vi "Coloured_Dot_Plotting.vi"(1 "JobVectorDirectory":path, 2 "Data":string[][](array[string]), 3 "Template Filename":path, 4 "Channel Names":string[](array[string])) -> ()   [LabVIEW 2015]
uses:
  Controls/Group_Binning.ctl
  Data_File_Type.ctl
panel:
  in  "Moving Z":u16(ring) items=["FF (C) X Position X (mm)", "FF (C) Y Position Y (mm)", "FF (C) Z Position Z (mm)", "FF (C) Mean C", "FF (C) Variance c^2", "EnFlo_Tunnel Source_Pos X", "EnFlo_Tunnel Source_Pos Y", "EnFlo_Tunnel Source_Pos Z", "EnFlo_Tunnel Reference Velocity", "GMU Trace Meas Q", "Multi Run Start Time", "Delta_x", "Delta_y", "Delta_z", "R", "User Comments", "EnFlo_Tunnel Source_Pos X_Model", "EnFlo_Tunnel Source_Pos Y_Model"]
  in  "Moving Y":u16(ring) items=["FF (C) X Position X (mm)", "FF (C) Y Position Y (mm)", "FF (C) Z Position Z (mm)", "FF (C) Mean C", "FF (C) Variance c^2", "EnFlo_Tunnel Source_Pos X", "EnFlo_Tunnel Source_Pos Y", "EnFlo_Tunnel Source_Pos Z", "EnFlo_Tunnel Reference Velocity", "GMU Trace Meas Q", "Multi Run Start Time", "Delta_x", "Delta_y", "Delta_z", "R", "User Comments", "EnFlo_Tunnel Source_Pos X_Model", "EnFlo_Tunnel Source_Pos Y_Model"]
  in  "Moving X":u16(ring) items=["FF (C) X Position X (mm)", "FF (C) Y Position Y (mm)", "FF (C) Z Position Z (mm)", "FF (C) Mean C", "FF (C) Variance c^2", "EnFlo_Tunnel Source_Pos X", "EnFlo_Tunnel Source_Pos Y", "EnFlo_Tunnel Source_Pos Z", "EnFlo_Tunnel Reference Velocity", "GMU Trace Meas Q", "Multi Run Start Time", "Delta_x", "Delta_y", "Delta_z", "R", "User Comments", "EnFlo_Tunnel Source_Pos X_Model", "EnFlo_Tunnel Source_Pos Y_Model"]
  in  "Scalar":u16(ring) items=["FF (C) X Position X (mm)", "FF (C) Y Position Y (mm)", "FF (C) Z Position Z (mm)", "FF (C) Mean C", "FF (C) Variance c^2", "EnFlo_Tunnel Source_Pos X", "EnFlo_Tunnel Source_Pos Y", "EnFlo_Tunnel Source_Pos Z", "EnFlo_Tunnel Reference Velocity", "GMU Trace Meas Q", "Multi Run Start Time", "Delta_x", "Delta_y", "Delta_z", "R", "User Comments", "EnFlo_Tunnel Source_Pos X_Model", "EnFlo_Tunnel Source_Pos Y_Model"]
  in  "Fixed Z":u16(ring) items=["FF (C) X Position X (mm)", "FF (C) Y Position Y (mm)", "FF (C) Z Position Z (mm)", "FF (C) Mean C", "FF (C) Variance c^2", "EnFlo_Tunnel Source_Pos X", "EnFlo_Tunnel Source_Pos Y", "EnFlo_Tunnel Source_Pos Z", "EnFlo_Tunnel Reference Velocity", "GMU Trace Meas Q", "Multi Run Start Time", "Delta_x", "Delta_y", "Delta_z", "R", "User Comments", "EnFlo_Tunnel Source_Pos X_Model", "EnFlo_Tunnel Source_Pos Y_Model"]
  in  "Fixed Y":u16(ring) items=["FF (C) X Position X (mm)", "FF (C) Y Position Y (mm)", "FF (C) Z Position Z (mm)", "FF (C) Mean C", "FF (C) Variance c^2", "EnFlo_Tunnel Source_Pos X", "EnFlo_Tunnel Source_Pos Y", "EnFlo_Tunnel Source_Pos Z", "EnFlo_Tunnel Reference Velocity", "GMU Trace Meas Q", "Multi Run Start Time", "Delta_x", "Delta_y", "Delta_z", "R", "User Comments", "EnFlo_Tunnel Source_Pos X_Model", "EnFlo_Tunnel Source_Pos Y_Model"]
  in  "Fixed X":u16(ring) items=["FF (C) X Position X (mm)", "FF (C) Y Position Y (mm)", "FF (C) Z Position Z (mm)", "FF (C) Mean C", "FF (C) Variance c^2", "EnFlo_Tunnel Source_Pos X", "EnFlo_Tunnel Source_Pos Y", "EnFlo_Tunnel Source_Pos Z", "EnFlo_Tunnel Reference Velocity", "GMU Trace Meas Q", "Multi Run Start Time", "Delta_x", "Delta_y", "Delta_z", "R", "User Comments", "EnFlo_Tunnel Source_Pos X_Model", "EnFlo_Tunnel Source_Pos Y_Model"]
  in  "OK Button":bool
  in  "Row Selector":i32(listbox)=1
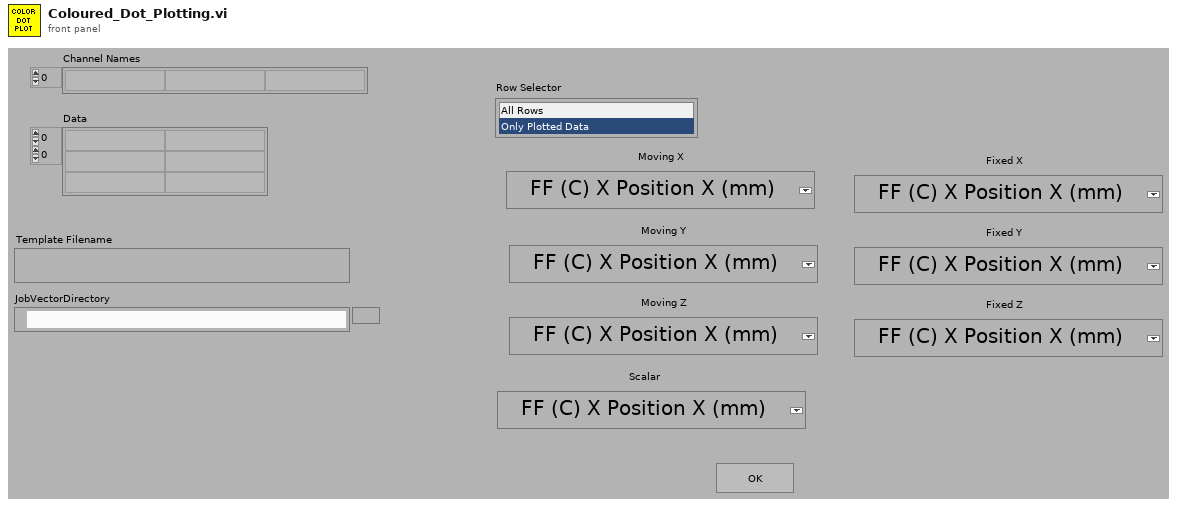
[diagram p1: front panel]
types:
  T1 = typedef "Data_File_Type.ctl" = enum16{"Read All File Types", "Results Files Only", "Raw Data Files Only", "Calibration Files Only", "Gas Desk Files Only", "Old Results Files Only", "Tabulated Data Files Only"}
  T2 = enum16{"Show only data summary", "Show data summary", "No data summary"}
  T3 = typedef "Group_Binning.ctl" = cluster{"Index":i32, "Tolerance":dbl, "Precision":string}
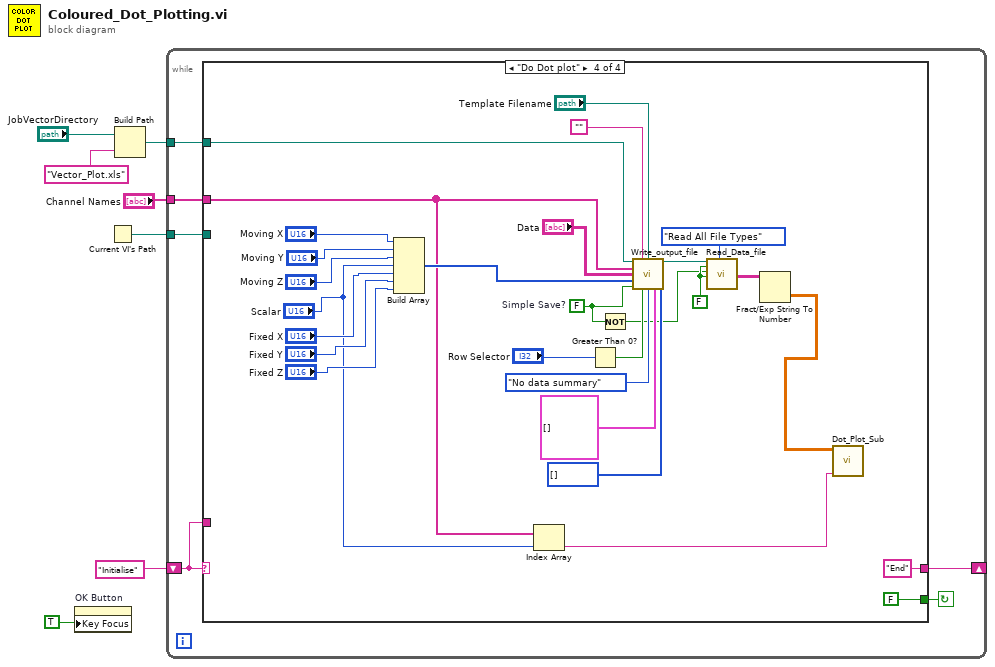
[diagram p0: block diagram]
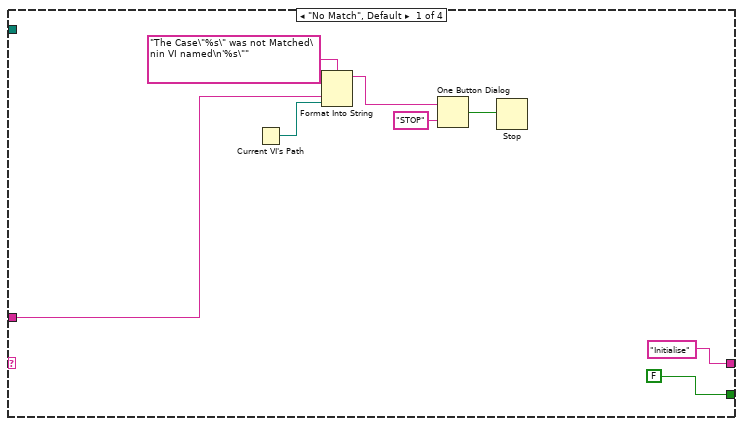
[diagram p2: hidden frame]
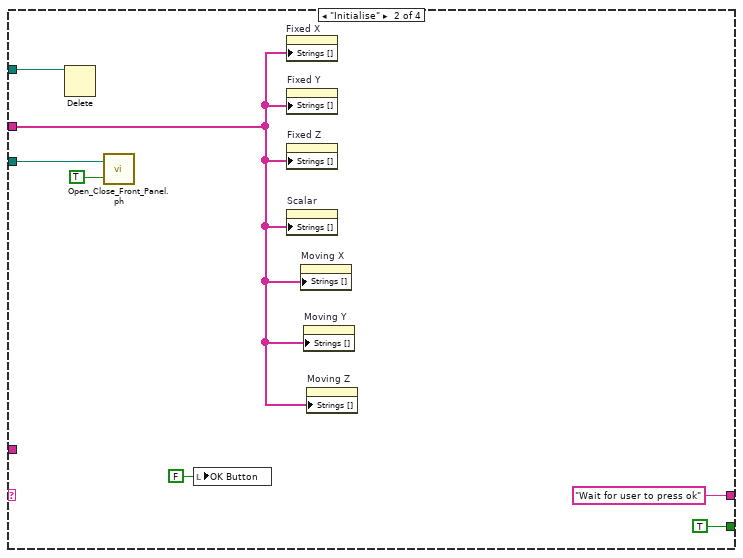
[diagram p3: hidden frame]
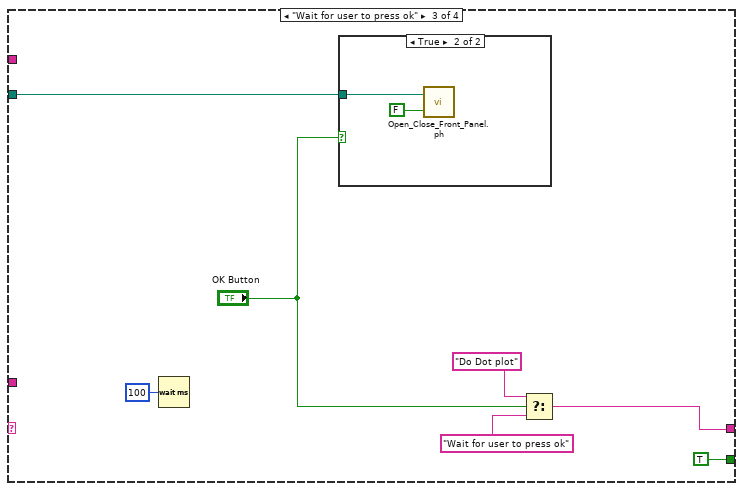
[diagram p4: hidden frame]
diagram:
  n1 = property on="OK Button" class="Bool (strict)"("Key Focus"=TRUE) -> ()  [unwired: 2 in, 2 out]
  n2 = Current VI's Path() -> (path=w6:path)
  n3 = Build Path(base path="JobVectorDirectory", name or relative path="Vector_Plot.xls") -> (appended path=w1:path)
  n4 = while {
    shift-left: "Initialise" -> [w11]
    shift-right: [w12] -> _
    tunnel: w6 -> [w10]
    tunnel: "Channel Names" -> [w9]
    tunnel: w1 -> [w8]
    stop <- w13 continue-if-true
    n5 = case shown="\"Do Dot plot\"" w11 {
      tunnel: [FALSE TRUE TRUE FALSE] -> w13
      tunnel: ["Initialise" "Wait for user to press ok" w34 "End" ("t")] -> w12
      tunnel: w11 -> [w16 _ _ _]
      tunnel: w10 -> [_ w26 w29 _]
      tunnel: w9 -> [_ w22 _ w43]
      tunnel: w8 -> [_ w23 _ w53]
      frame "No Match", Default {
        n6 = Current VI's Path() -> (path=w15:path)
        n7 = Format Into String(format string="The Case\"%s\" was not Matched\nin VI named\n'%s\"" ("Format String"), w16, w15) -> (resulting string=w19:string)  [unwired: 2 in, 1 out]
        n8 = One Button Dialog(message=w19, button name ("OK")="STOP") -> (true=w17:bool)
        n9 = Stop(stop? (T)=w17) -> ()
      }
      frame "Initialise" {
        n10 = Delete(path (use dialog)=w23) -> ()  [unwired: 1 in, 6 out]
        n11 = call "Open_Close_Front_Panel.ph.vi"("Front Panel Window:Open"=TRUE, "VI path"=w26) -> ()  [unwired: 2 out]
        n12 = local write "OK Button"(FALSE ("OK Button")) -> ()
        n13 = property on="Fixed X" class="Ring (strict)"("Strings []"=w22) -> ()  [unwired: 2 in, 2 out]
        n14 = property on="Fixed Y" class="Ring (strict)"("Strings []"=w22) -> ()  [unwired: 2 in, 2 out]
        n15 = property on="Fixed Z" class="Ring (strict)"("Strings []"=w22) -> ()  [unwired: 2 in, 2 out]
        n16 = property on="Scalar" class="Ring (strict)"("Strings []"=w22) -> ()  [unwired: 2 in, 2 out]
        n17 = property on="Moving X" class="Ring (strict)"("Strings []"=w22) -> ()  [unwired: 2 in, 2 out]
        n18 = property on="Moving Y" class="Ring (strict)"("Strings []"=w22) -> ()  [unwired: 2 in, 2 out]
        n19 = property on="Moving Z" class="Ring (strict)"("Strings []"=w22) -> ()  [unwired: 2 in, 2 out]
      }
      frame "Wait for user to press ok" {
        n20 = Wait (ms)(milliseconds to wait=u32 100) -> ()  [unwired: 1 out]
        n21 = case shown="True" "OK Button" {
          tunnel: w29 -> [_ w36]
          frame False {
          }
          frame True {
            n22 = call "Open_Close_Front_Panel.ph.vi"("Front Panel Window:Open"=FALSE, "VI path"=w36) -> ()  [unwired: 2 out]
          }
        }
        n23 = Select(t="Do Dot plot", s="OK Button", f="Wait for user to press ok") -> (s? t:f=w34:string)
      }
      frame "Do Dot plot" {
        w56 = FALSE ("Read Channel Names only")
        w40 = FALSE  # Simple Save?
        n24 = Build Array("Moving X", "Moving Y", "Moving Z", "Scalar", "Fixed X", "Fixed Y", "Fixed Z") -> (w44:u16[])
        n25 = Index Array(array=w43, index="Scalar") -> (element=w41:string)
        n26 = Greater Than 0?(x="Row Selector") -> (x > 0?=w59:bool)
        n27 = Not(x=w40) -> (.not. x?=w39:bool)
        n28 = call "Write_output_file.vi"("Output filename"=w53, "Header"="", "Template Filename"="Template Filename", "Channel Names"=w43, "Data"="Data", "Desired Columns"=w44, "Simple Save?"=w40, "Save Plotted rows only?"=w59, "Summarise mode"=T2."No data summary", "Grouping info"=T3[] [], "Channels to Tabulate in header"=i32[] []) -> ("Output filename Out"=w51:path)  [unwired: 1 in, 3 out]
        n29 = call "Read_Data_file.vi"("Results file"=w51, "Read Channel Names only"=w56, "Delete First Rows?"=w39, "Add Extra Channels?"=w56, "Desired File Types"=Data_File_Type."Read All File Types") -> ("Channel Values Out"=w54:string[][])  [unwired: 1 in, 13 out]
        n30 = Fract/Exp String To Number(string=w54) -> (number=w38:dbl[][])  [unwired: 4 out]
        n31 = call "Dot_Plot_Sub.vi"("Scaler plotted"=w41, "Data"=w38) -> ()  [unwired: 10 in]
      }
    }
  }
